vi "DHE_MacroPreProc.vi"(9 "args":string[](array[string]), 10 "cmds in":string) -> (1 "args out":string[](array[string]), 2 "cmd out":string)   [LabVIEW 2016]
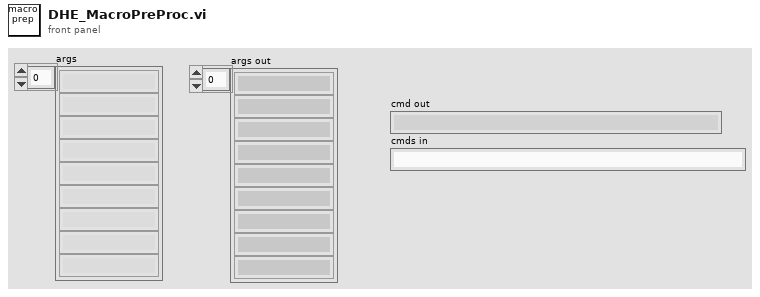
[diagram p1: front panel]
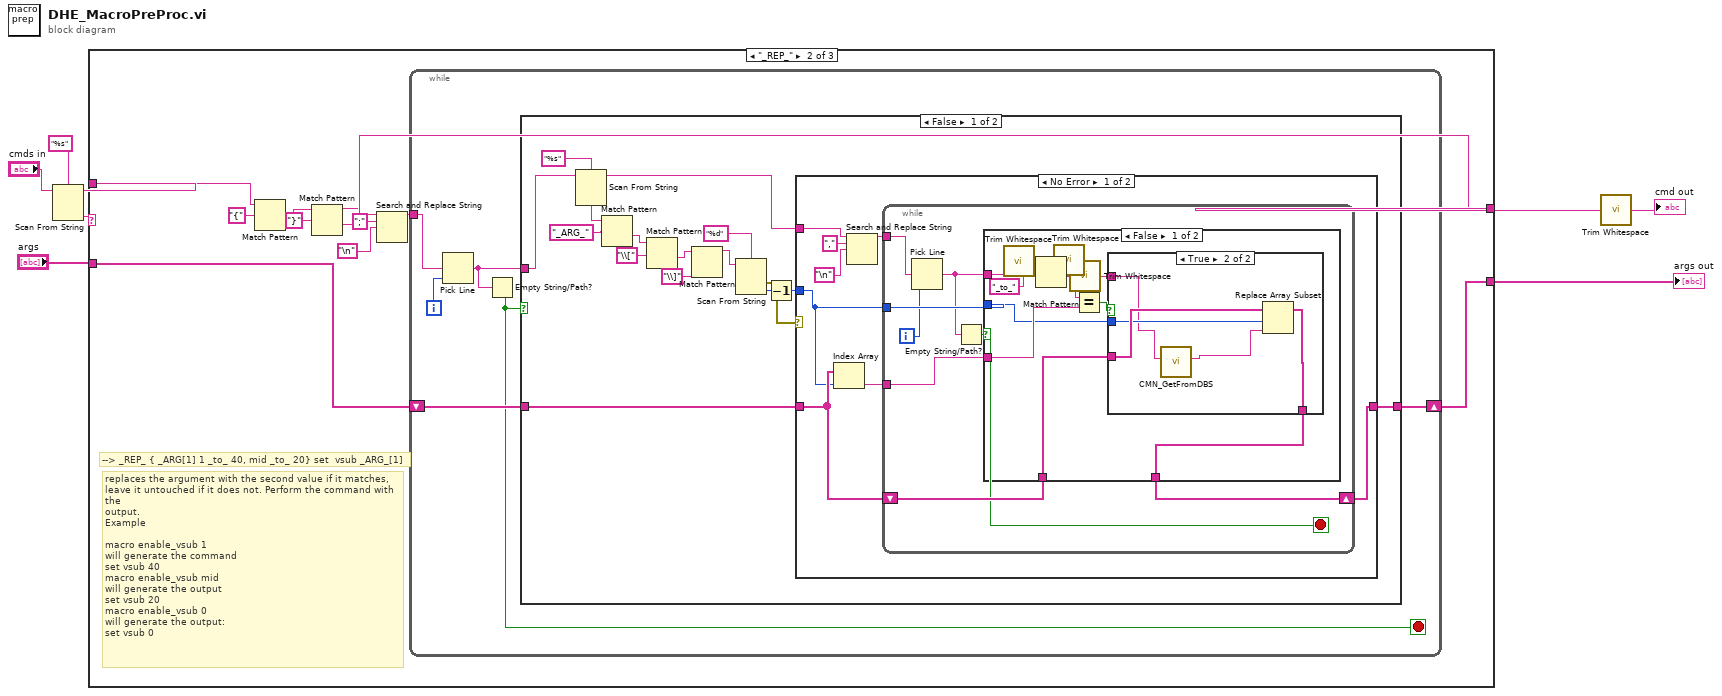
[diagram p0: block diagram]
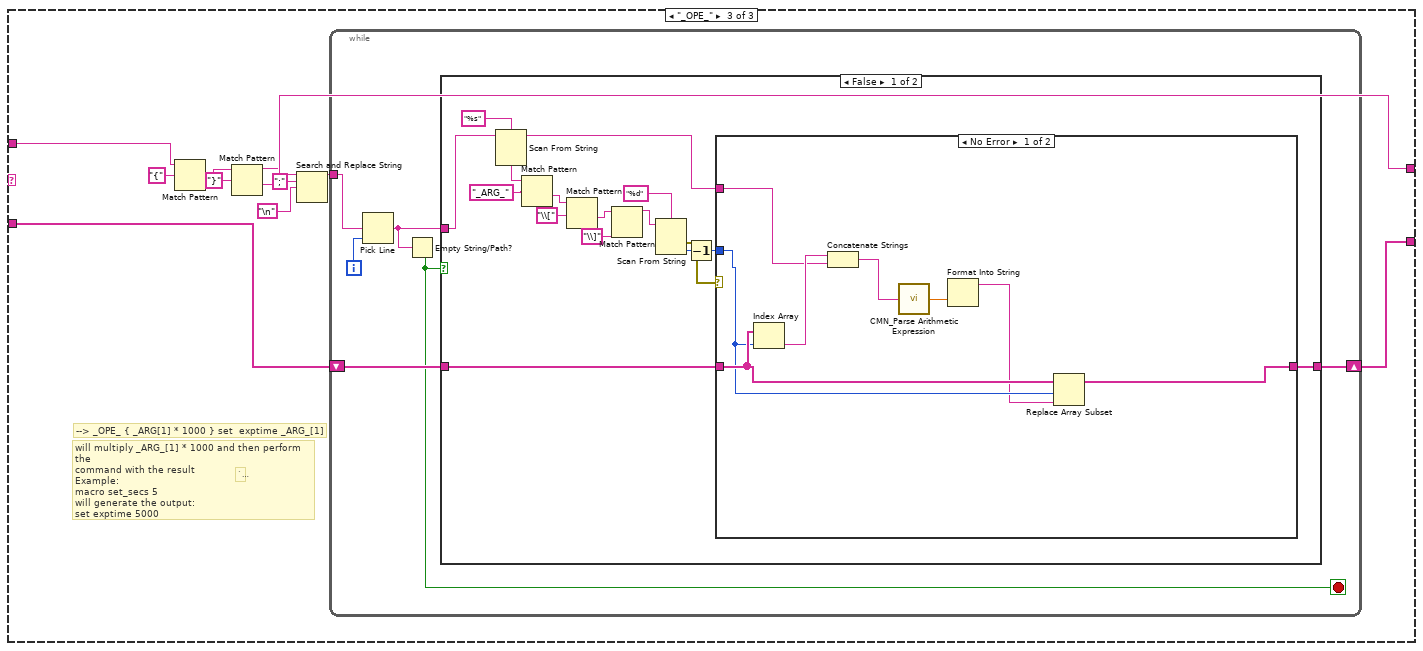
[diagram p7: hidden frame]
diagram:
  n1 = Scan From String(format string="%s", input string="cmds in") -> (remaining string=w3:string, output 1=w2:string)  [unwired: 2 in, 3 out]
  n2 = case shown="\"_REP_\"" w2 {
    tunnel: [w10 w21 w91] -> w8
    tunnel: [w9 w15 w85] -> w7
    tunnel: "args" -> [w10 w20 w90]
    tunnel: w3 -> [w9 w19 w89]
    frame Default {
    }
    frame "_REP_" {
      # "replaces the argument with the second value if it matches,\nleave it untouched if it does not. Perform the command with the\noutput.\nExample\n\nmacro enable_vsub 1\nwill generate the command\nset vsub 40\nmacro enable_vsub mid\nwill generate the output\nset vsub 20\nmacro enable_vsub 0\nwill generate the output:\nset vsub 0"
      # "--> _REP_ { _ARG[1] 1 _to_ 40, mid _to_ 20} set  vsub _ARG_[1]"
      n3 = Match Pattern(string=w19, regular expression="{") -> (after substring=w17:string)  [unwired: 4 out]
      n4 = Match Pattern(string=w17, regular expression="}") -> (before substring=w14:string, after substring=w15:string)  [unwired: 3 out]
      n5 = Search and Replace String(input string=w14, search string=";", replace string="\n") -> (result string=w11:string)  [unwired: 5 in, 3 out]
      n6 = while {
        shift-right: [w27] -> w21
        shift-left: w20 -> [w26]
        tunnel: w11 -> [w22]
        i -> [w25]
        stop <- w23 stop-if-true
        n7 = Pick Line(multi-line string=w22, line index=w25) -> (output string=w24:string)  [unwired: 1 in]
        n8 = Empty String/Path?(string/path=w24) -> (empty?=w23:bool)
        n9 = case shown="False" w23 {
          tunnel: [w33 w80] -> w27
          tunnel: w26 -> [w30 w80]
          tunnel: w24 -> [w29 _]
          frame False {
            n10 = Scan From String(format string="%s", input string=w29) -> (remaining string=w32:string, output 1=w41:string)  [unwired: 2 in, 3 out]
            n11 = Match Pattern(string=w41, regular expression="_ARG_") -> (after substring=w40:string)  [unwired: 4 out]
            n12 = Match Pattern(string=w40, regular expression="\\[") -> (after substring=w38:string)  [unwired: 4 out]
            n13 = Match Pattern(string=w38, regular expression="\\]") -> (before substring=w36:string)  [unwired: 4 out]
            n14 = Scan From String(format string="%d", input string=w36) -> (error out=w34:errorcluster, output 1=w31:i32)  [unwired: 2 in, 3 out]
            n15 = Decrement(x=w31) -> (x-1=w28:i32)
            n16 = case shown="No Error" w34 {
              tunnel: w30 -> [w46 w79]
              tunnel: [w51 w79] -> w33
              tunnel: w32 -> [w50 _]
              tunnel: w28 -> [w45 _]
              frame No Error {
                n17 = Index Array(array=w46, index=w45) -> (element=w44:string)
                n18 = Search and Replace String(input string=w50, search string=",", replace string="\n") -> (result string=w47:string)  [unwired: 5 in, 3 out]
                n19 = while {
                  tunnel: w45 -> [w57]
                  shift-right: [w58] -> w51
                  shift-left: w46 -> [w59]
                  tunnel: w47 -> [w52]
                  tunnel: w44 -> [w53]
                  i -> [w56]
                  stop <- w55 stop-if-true
                  n20 = Pick Line(multi-line string=w52, line index=w56) -> (output string=w54:string)  [unwired: 1 in]
                  n21 = Empty String/Path?(string/path=w54) -> (empty?=w55:bool)
                  n22 = case shown="False" w55 {
                    tunnel: w59 -> [w67 w78]
                    tunnel: [w66 w78] -> w58
                    tunnel: w57 -> [w65 _]
                    tunnel: w54 -> [w71 _]
                    tunnel: w53 -> [w69 _]
                    frame False {
                      n23 = call <vilib>:"Trim Whitespace.vi"("string"=w71) -> ("trimmed string"=w64:string)  [unwired: 1 in]
                      n24 = Match Pattern(string=w64, regular expression="_to_") -> (before substring=w62:string, after substring=w63:string)  [unwired: 3 out]
                      n25 = call <vilib>:"Trim Whitespace.vi"("string"=w62) -> ("trimmed string"=w61:string)  [unwired: 1 in]
                      n26 = call <vilib>:"Trim Whitespace.vi"("string"=w63) -> ("trimmed string"=w60:string)  [unwired: 1 in]
                      n27 = Equal?(x=w61, y=w69) -> (x = y?=w68:bool)
                      n28 = case shown="True" w68 {
                        tunnel: w60 -> [_ w74]
                        tunnel: w67 -> [w72 w77]
                        tunnel: [w72 w75] -> w66
                        tunnel: w65 -> [_ w76]
                        frame False {
                        }
                        frame True {
                          n29 = call "CMN_GetFromDBS.vi"("str in"=w74) -> ("str out"=w73:string)  [unwired: 10 in]
                          n30 = Replace Array Subset(array=w77, new element=w73, index=w76) -> (w75:string[])
                        }
                      }
                    }
                    frame True {
                    }
                  }
                }
              }
              frame Error {
              }
            }
          }
          frame True {
          }
        }
      }
    }
    frame "_OPE_" {
      # "will multiply _ARG_[1] * 1000 and then perform the\ncommand with the result\nExample:\nmacro set_secs 5\nwill generate the output:\nset exptime 5000"
      # "``"
      # "--> _OPE_ { _ARG[1] * 1000 } set  exptime _ARG_[1]"
      n31 = Match Pattern(string=w89, regular expression="{") -> (after substring=w87:string)  [unwired: 4 out]
      n32 = Match Pattern(string=w87, regular expression="}") -> (before substring=w84:string, after substring=w85:string)  [unwired: 3 out]
      n33 = Search and Replace String(input string=w84, search string=";", replace string="\n") -> (result string=w81:string)  [unwired: 5 in, 3 out]
      n34 = while {
        shift-right: [w97] -> w91
        shift-left: w90 -> [w96]
        tunnel: w81 -> [w92]
        i -> [w95]
        stop <- w93 stop-if-true
        n35 = Pick Line(multi-line string=w92, line index=w95) -> (output string=w94:string)  [unwired: 1 in]
        n36 = Empty String/Path?(string/path=w94) -> (empty?=w93:bool)
        n37 = case shown="False" w93 {
          tunnel: [w103 w123] -> w97
          tunnel: w96 -> [w100 w123]
          tunnel: w94 -> [w99 _]
          frame False {
            n38 = Scan From String(format string="%s", input string=w99) -> (remaining string=w102:string, output 1=w111:string)  [unwired: 2 in, 3 out]
            n39 = Match Pattern(string=w111, regular expression="_ARG_") -> (after substring=w110:string)  [unwired: 4 out]
            n40 = Match Pattern(string=w110, regular expression="\\[") -> (after substring=w108:string)  [unwired: 4 out]
            n41 = Match Pattern(string=w108, regular expression="\\]") -> (before substring=w106:string)  [unwired: 4 out]
            n42 = Scan From String(format string="%d", input string=w106) -> (error out=w104:errorcluster, output 1=w101:i32)  [unwired: 2 in, 3 out]
            n43 = Decrement(x=w101) -> (x-1=w98:i32)
            n44 = case shown="No Error" w104 {
              tunnel: w100 -> [w118 w122]
              tunnel: [w114 w122] -> w103
              tunnel: w102 -> [w120 _]
              tunnel: w98 -> [w117 _]
              frame No Error {
                n45 = Index Array(array=w118, index=w117) -> (element=w121:string)
                n46 = Concatenate Strings(w121, w120) -> (w119:string)
                n47 = call "CMN_Parse Arithmetic Expression.vi"("Arithmetic Expression"=w119) -> ("Result"=w116:dbl)
                n48 = Format Into String(w116) -> (resulting string=w115:string)  [unwired: 3 in, 1 out]
                n49 = Replace Array Subset(array=w118, new element=w115, index=w117) -> (w114:string[])
              }
              frame Error {
              }
            }
          }
          frame True {
          }
        }
      }
    }
  }
  "args out" <- w8
  n50 = call <vilib>:"Trim Whitespace.vi"("string"=w7) -> ("trimmed string"=→"cmd out":string)  [unwired: 1 in]
